vi "探测器列表-加载全部.vi"(7 "table-探测器列表名":string="探测器列表", 8 "error in (no error)":errorcluster, 11 "数据库引用":T1) -> (0 "error out":errorcluster, 2 "探测器清单":T2[](array[typedef]), 3 "connection reference out":T1)   [LabVIEW 2017]
uses:
  <vilib>/addons/database/Connection.llb/Conn ObjectReference.ctl
  <vilib>/addons/database/_DB Variant To Data/Database Variant To Data.xnode
  <vilib>/addons/database/NI_Database_API.lvlib
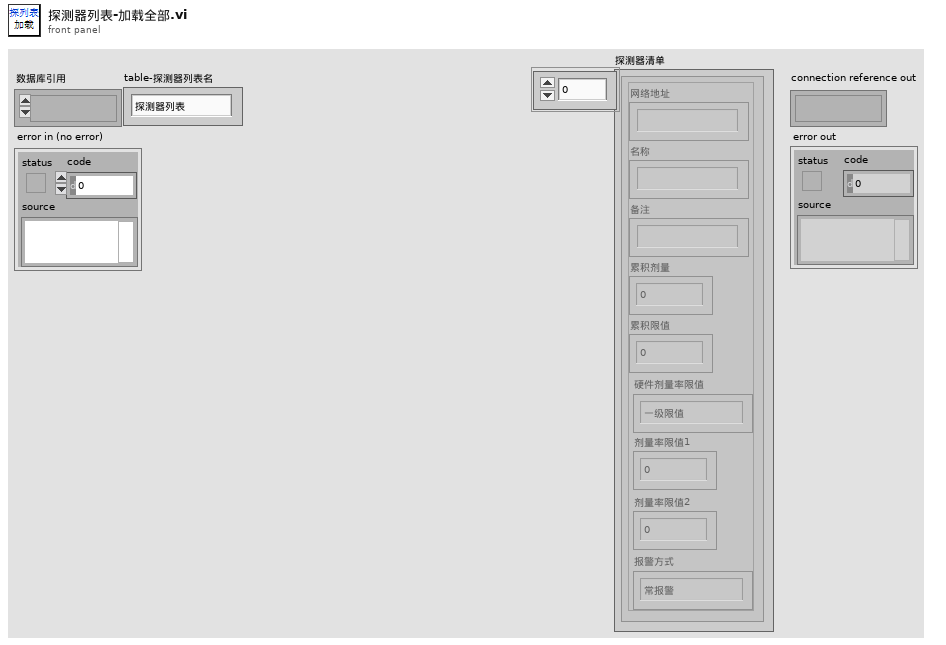
[diagram p1: front panel]
types:
  T1 = typedef "NI_Database_API.lvlib/Conn ObjectReference.ctl" = refnum<k1>
  T2 = typedef "探测器信息.ctl" = cluster{"网络地址":string, "名称":string, "备注":string, "累积剂量":dbl, "累积限值":dbl, "硬件剂量率限值":T3, "剂量率限值1":dbl, "剂量率限值2":dbl, "报警方式":T4}
  T3 = typedef "探头剂量率限值选择.ctl" = enum16{"一级限值", "二级限值"}
  T4 = typedef "报警方式选择.ctl" = enum16{"常报警", "自动静音", "手动静音"}
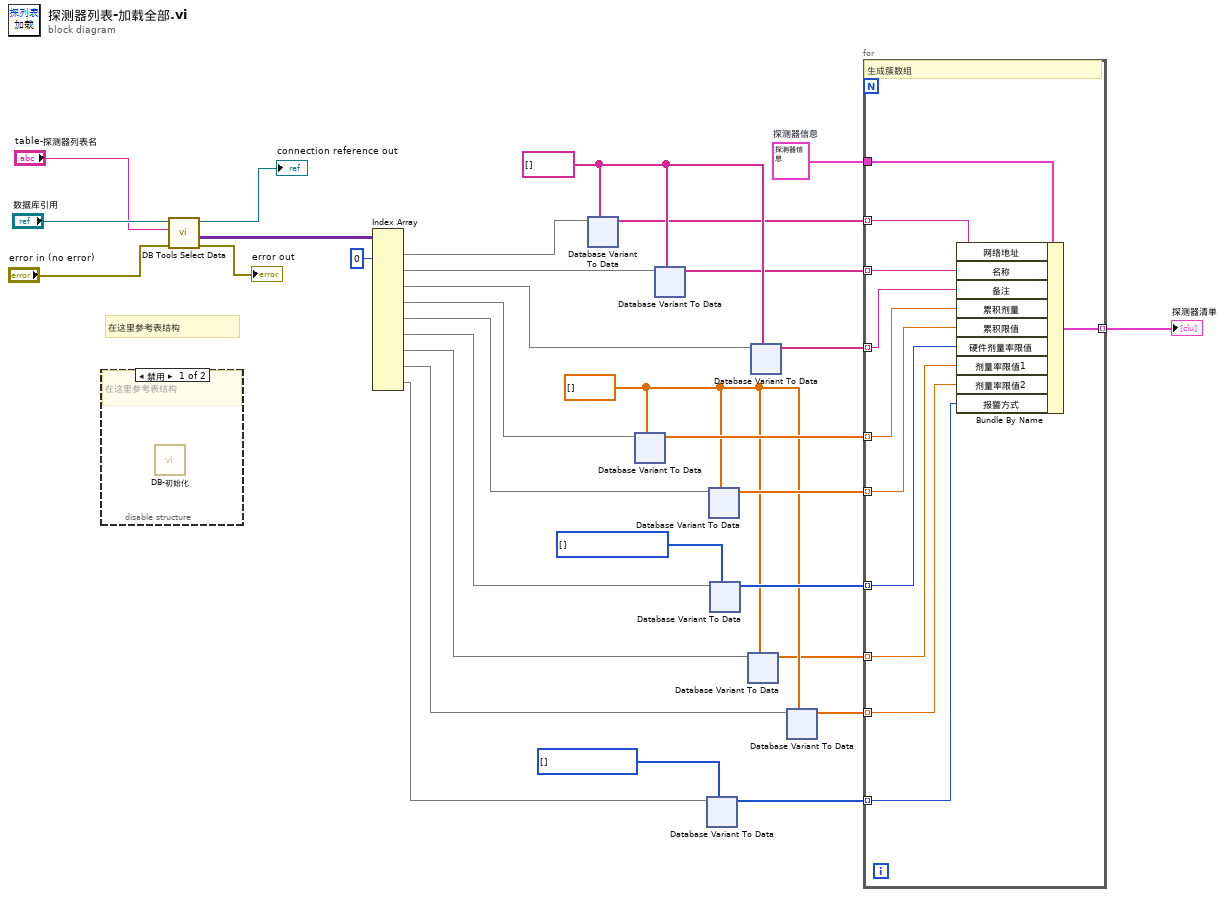
[diagram p0: block diagram]
diagram:
  w6 = T4[] [] items=["常报警", "自动静音", "手动静音"] ("报警方式")
  w7 = T3[] [] items=["一级限值", "二级限值"] ("硬件剂量率限值")
  w16 = T2 {"网络地址"="", "名称"="", "备注"="", "累积剂量"=0.0, "累积限值"=0.0, "硬件剂量率限值"=enum."一级限值", "剂量率限值1"=0.0, "剂量率限值2"=0.0, "报警方式"=enum."常报警"}  # 探测器信息
  w3 = dbl[] []
  w22 = string[] []
  # "在这里参考表结构"
  n1 = disable-structure shown="禁用" {
    frame Disabled {
      # "在这里参考表结构"
      n2 = call "DB-初始化.vi"() -> ()  [unwired: 10 in, 2 out]
    }
    frame Enabled {
    }
  }
  n3 = call <vilib>:"DB Tools Select Data.vi"("error in (no error)"="error in (no error)", "table"="table-探测器列表名", "connection reference"="数据库引用") -> ("error out"=→"error out":errorcluster, "data"=w29:variant[][], "connection reference out"=→"connection reference out":T1)  [unwired: 3 in]
  n4 = Index Array(array=w29, index (col) #1=0 ("禁用的索引 (列)")) -> (element #1=w27:variant[], element #2=w26:variant[], element #3=w25:variant[], element #4=w24:variant[], element #5=w23:variant[], element #6=w11:variant[], element #7=w10:variant[], element #8=w9:variant[], element #9=w8:variant[])  [unwired: 17 in]
  n5 = xnode "Database Variant To Data"("database variant"=w27, "type"=w22) -> ("data"=w21:string[])  [unwired: 1 in, 1 out]
  n6 = xnode "Database Variant To Data"("database variant"=w24, "type"=w3) -> ("data"=w18:dbl[])  [unwired: 1 in, 1 out]
  n7 = xnode "Database Variant To Data"("database variant"=w26, "type"=w22) -> ("data"=w20:string[])  [unwired: 1 in, 1 out]
  n8 = xnode "Database Variant To Data"("database variant"=w8, "type"=w6) -> ("data"=w4:T4[])  [unwired: 1 in, 1 out]
  n9 = xnode "Database Variant To Data"("database variant"=w23, "type"=w3) -> ("data"=w17:dbl[])  [unwired: 1 in, 1 out]
  n10 = xnode "Database Variant To Data"("database variant"=w11, "type"=w7) -> ("data"=w5:T3[])  [unwired: 1 in, 1 out]
  n11 = xnode "Database Variant To Data"("database variant"=w10, "type"=w3) -> ("data"=w2:dbl[])  [unwired: 1 in, 1 out]
  n12 = xnode "Database Variant To Data"("database variant"=w25, "type"=w22) -> ("data"=w19:string[])  [unwired: 1 in, 1 out]
  n13 = xnode "Database Variant To Data"("database variant"=w9, "type"=w3) -> ("data"=w1:dbl[])  [unwired: 1 in, 1 out]
  n14 = for {
    tunnel: w21 -> [w41] mode=indexing
    tunnel: w20 -> [w40] mode=indexing
    tunnel: w19 -> [w39] mode=indexing
    tunnel: w18 -> [w38] mode=indexing
    tunnel: w17 -> [w37] mode=indexing
    tunnel: w16 -> [w42]
    tunnel: [w36] -> w15 mode=indexing
    tunnel: w5 -> [w35] mode=indexing
    tunnel: w4 -> [w34] mode=indexing
    tunnel: w2 -> [w33] mode=indexing
    tunnel: w1 -> [w32] mode=indexing
    # "生成簇数组"
    n15 = Bundle By Name(cluster=w42, "网络地址"=w41, "名称"=w40, "备注"=w39, "累积剂量"=w38, "累积限值"=w37, "硬件剂量率限值"=w35, "剂量率限值1"=w33, "剂量率限值2"=w32, "报警方式"=w34) -> (w36:T2)
  }
  "探测器清单" <- w15
